vi "svc_Get Continuous Data Subset.vi"(7 "restart":bool, 9 "block size (samples)":i32, 10 "start index":i32, 11 "signal in":waveform(dbl)) -> (1 "new data available":bool, 3 "subset out":waveform(dbl))   [LabVIEW 2017]
uses:
  <vilib>/addons/_NISVFA/_Shared subVIs/Common/svc_Check for Waveform Parameter Continuity (no state).vi
  <vilib>/addons/_NISVFA/_Shared subVIs/Common/svc_Get SV Channel Info.vi
  <vilib>/Waveform/WDTOps.llb/WDT Get Waveform Subset DBL.vi
  <vilib>/Waveform/WDTOps.llb/WDT Append Waveforms DBL.vi
  <vilib>/addons/_NISVFA/_Shared subVIs/Common/svc_Engineering Units to Unit Label.vi
  <vilib>/addons/_NISVFA/_Shared subVIs/Common/svc_Unit Label to Engineering Units.vi
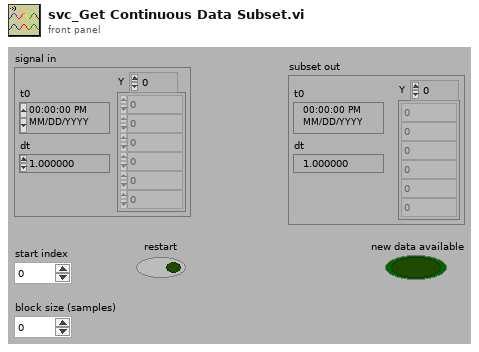
[diagram p1: front panel]
types:
  T1 = cluster{"ignore dt":bool, "ignore t0 continuity":bool, "ignore array length":bool, "ignore channel info":bool, "ignore channel name":bool}
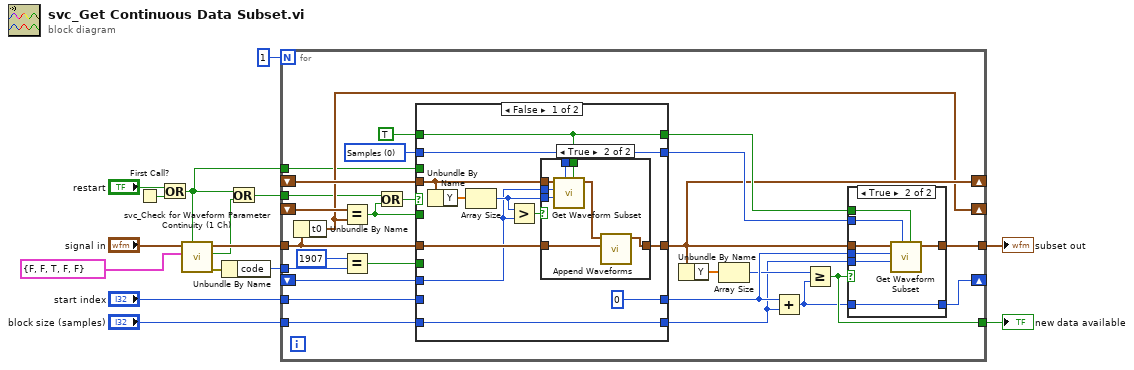
[diagram p0: block diagram]
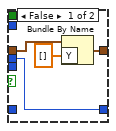
[diagram p2: hidden frame]
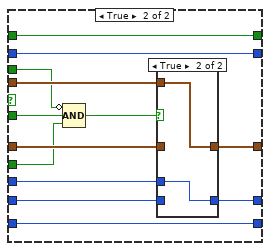
[diagram p4: hidden frame]
diagram:
  n1 = First Call?() -> (First Call?: T/F=w1:bool)
  n2 = Or(x="restart", y=w1) -> (x .or. y?=w2:bool)
  n3 = call <vilib>:"svc_Check for Waveform Parameter Continuity (1 Ch).vi"("restart averaging (F)"=w2, "checks for channel parameter change"=T1 {"ignore dt"=FALSE, "ignore t0 continuity"=FALSE, "ignore array length"=TRUE, "ignore channel info"=FALSE, "ignore channel name"=FALSE} ("parameter controls"), "scaled signal [EU]"="signal in") -> ("error out"=w4:errorcluster, "waveform parameter changed"=w7:bool, "dup scaled signal [EU]"=w10:waveform(dbl))  [unwired: 3 in, 3 out]
  n4 = Unbundle By Name(w4) -> ("code"=w3:i32)
  n5 = Or(x=w2, y=w7) -> (x .or. y?=w8:bool)
  n6 = for {
    N: 1 -> [_]
    tunnel: "block size (samples)" -> [w27]
    shift-right: [w25] -> _
    shift-left: _ -> [w42]
    tunnel: [w34] -> w5
    tunnel: w10 -> [w38]
    tunnel: w8 -> [w22]
    tunnel: "start index" -> [w40]
    shift-right: [w16] -> _
    shift-left: _ -> [w36]
    shift-right: [w23] -> _
    shift-left: _ -> [w39]
    tunnel: [w28] -> w6
    tunnel: w3 -> [w21]
    tunnel: w2 -> [w18]
    w32 = u16 0 items=["Samples", "Relative Time"] ("start/duration format")
    n7 = Unbundle By Name(w38) -> ("t0"=w23:timestamp)
    n8 = Equal?(x=w39, y=w23) -> (x = y?=w24:bool)
    n9 = Equal?(x=1907, y=w21) -> (x = y?=w19:bool)
    n10 = Or(x=w22, y=w24) -> (x .or. y?=w37:bool)
    n11 = case shown="False" w37 {
      tunnel: w42 -> [w57 w80]
      tunnel: w38 -> [w64 w79]
      tunnel: [w63 w78] -> w25
      tunnel: w40 -> [_ w83]
      tunnel: [0 ("start index") w82] -> w35
      tunnel: w36 -> [w55 w81]
      tunnel: w32 -> [w61 w85]
      tunnel: TRUE ("open interval? (T)") -> [w60 w86]
      tunnel: [w60 w86] -> w30
      tunnel: [w61 w85] -> w29
      tunnel: w27 -> [w59 w84]
      tunnel: [w59 w84] -> w26
      tunnel: w24 -> [_ w77]
      tunnel: w19 -> [_ w76]
      tunnel: w18 -> [_ w74]
      frame False {
        n12 = Unbundle By Name(w57) -> ("Y"=w58:dbl[])
        n13 = Array Size(array=w58) -> (size(s)=w56:i32)
        n14 = Greater?(x=w56, y=w55) -> (0:w54:bool)
        n15 = case shown="True" w54 {
          tunnel: w64 -> [w65 w73]
          tunnel: [w65 w72] -> w63
          tunnel: w55 -> [_ w70]
          tunnel: w61 -> [_ w69]
          tunnel: w60 -> [_ w68]
          tunnel: w57 -> [_ w67]
          tunnel: w56 -> [_ w66]
          frame False {
          }
          frame True {
            n16 = call-poly <vilib>:"Get Waveform Subset.vi"("open interval? (T)"=w68, "start/duration format"=w69, "duration"=w66, "start samples/time"=w70, "waveform in"=w67) -> ("waveform out"=w71:waveform(dbl))  [unwired: 1 in, 3 out]
            n17 = call-poly <vilib>:"Append Waveforms.vi"("waveform B"=w73, "waveform A"=w71) -> ("waveform out"=w72:waveform(dbl))  [unwired: 8 in, 1 out]
          }
        }
      }
      frame True {
        n18 = Compound Arithmetic op=AND(invert w74, w77, w76) -> (w75:bool)
        n19 = case shown="True" w75 {
          tunnel: w83 -> [w88 _]
          tunnel: [w88 w90] -> w82
          tunnel: w81 -> [_ w90]
          tunnel: w80 -> [_ w89]
          tunnel: w79 -> [w87 _]
          tunnel: [w87 w89] -> w78
          frame False {
          }
          frame True {
          }
        }
      }
    }
    n20 = Unbundle By Name(w25) -> ("Y"=w41:dbl[])
    n21 = Array Size(array=w41) -> (size(s)=w33:i32)
    n22 = Add(x=w35, y=w26) -> (x+y=w17:i32)
    n23 = Greater Or Equal?(x=w33, y=w17) -> (x >= y?=w28:bool)
    n24 = case shown="True" w28 {
      tunnel: w35 -> [w43 w53]
      tunnel: w26 -> [_ w52]
      tunnel: [w45 w51] -> w34
      tunnel: w25 -> [w46 w50]
      tunnel: w30 -> [_ w49]
      tunnel: w29 -> [_ w48]
      tunnel: w17 -> [_ w47]
      tunnel: [w43 w47] -> w16
      frame False {
        n25 = Bundle By Name(cluster=w46, "Y"=dbl[] []) -> (w45:waveform(dbl))
      }
      frame True {
        n26 = call-poly <vilib>:"Get Waveform Subset.vi"("open interval? (T)"=w49, "start/duration format"=w48, "duration"=w52, "start samples/time"=w53, "waveform in"=w50) -> ("waveform out"=w51:waveform(dbl))  [unwired: 1 in, 3 out]
      }
    }
  }
  "subset out" <- w5
  "new data available" <- w6
